vi "Read.vi"(8 "error in (no error)":errorcluster, 11 "WebSocket in":refnum<class "WebSocket.lvclass">) -> (0 "error out":errorcluster, 3 "WebSocket out":refnum<class "WebSocket.lvclass">)   [LabVIEW 2021, in "WebSocket.lvlib" / "WebSocket.lvclass"]
uses:
  WebSocket.lvclass
  C:/Program Files (x86)/National Instruments/LabVIEW 2021/vi.lib/ActorFramework/Actor/Actor.lvclass
  WebSocket.lvclass/WebSocket.ctl
  <vilib>/ActorFramework/Actor/Actor.lvclass/Actor.ctl
  <vilib>/ActorFramework/Message Enqueuer/Message Enqueuer.lvclass/Message Enqueuer.ctl
  <vilib>/ActorFramework/Message Enqueuer/Init from Existing Queue.vi
  <vilib>/ActorFramework/Message Enqueuer/Enqueue.vi
  WebSocket Messages/Read Msg/Read Msg.lvclass
  C:/Program Files (x86)/National Instruments/LabVIEW 2021/vi.lib/ActorFramework/Message/Message.lvclass
  WebSocket Messages/WaitListener Msg/WaitListener Msg.lvclass
  <vilib>/ActorFramework/Message Priority Queue/Priority Enqueue.vi
  <vilib>/ActorFramework/Message Enqueuer/Message Enqueuer.lvclass
  <vilib>/MediaMongrels Ltd/WebSockets/WebSockets/WebSocket Server/WebSocket Server.lvclass
  <vilib>/ActorFramework/Actor/Actor.lvclass
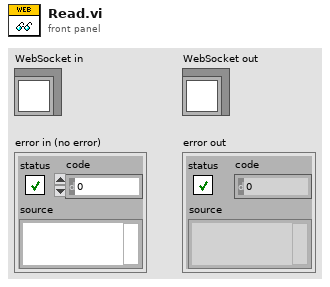
[diagram p1: front panel]
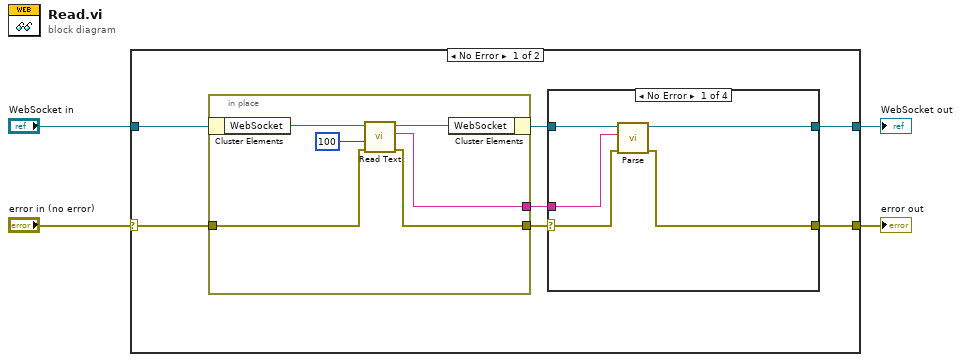
[diagram p0: block diagram]
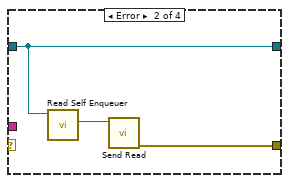
[diagram p2: hidden frame]
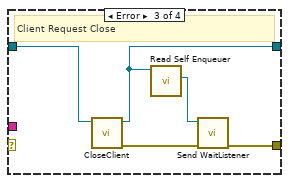
[diagram p3: hidden frame]
diagram:
  n1 = case shown="No Error" "error in (no error)" {
    selector: "error in (no error)" -> [w10 w34]
    tunnel: [w5 w34] -> w3
    tunnel: [w8 w33] -> w1
    tunnel: "WebSocket in" -> [w11 w33]
    frame No Error {
      n2 = in-place {
        in-place-border: w10 -> [w29]
        in-place-border: [w28] -> w6
        in-place-border: [w27] -> w7
        n3 = in-place-cluster #1(w11) -> ("WebSocket"=w31:refnum<class "WebSocket Server.lvclass">)
        n4 = call-dynamic "Read Text.vi"("error in (no error)"=w29, "timeout ms (5000)"=100 ("timeout ms (25000)"), "WebSocket in"=w31) -> ("error out"=w28:errorcluster, "Data"=w27:string, "WebSocket out"=w30:refnum<class "WebSocket Server.lvclass">)  [unwired: 6 in]
        n5 = in-place-cluster #1("WebSocket"=w30) -> (w9:refnum<class "WebSocket.lvclass">)
      }
      n6 = case shown="No Error" w6 {
        selector: w6 -> [w12 _ _ w25]
        tunnel: w9 -> [w16 w19 w24 w26]
        tunnel: [w15 w19 w20 w26] -> w8
        tunnel: w7 -> [w14 _ _ _]
        tunnel: [w13 w17 w21 w25] -> w5
        frame No Error {
          n7 = call "Parse.vi"("error in (no error)"=w12, "Data"=w14, "WebSocket in"=w16) -> ("error out"=w13:errorcluster, "WebSocket out"=w15:refnum<class "WebSocket.lvclass">)  [unwired: 7 in]
        }
        frame Error {
          n8 = call <vilib>:"Read Self Enqueuer.vi"("Actor"=w19) -> ("Self Enqueuer"=w18:refnum<class "Message Enqueuer.lvclass">)  [unwired: 10 in]
          n9 = call "Send Read.vi"("Message Enqueuer"=w18) -> ("error out"=w17:errorcluster)  [unwired: 9 in, 1 out]
        }
        frame Error {
          # "Client Request Close"
          n10 = call "CloseClient.vi"("WebSocket in"=w24) -> ("error out"=w22:errorcluster, "WebSocket out"=w20:refnum<class "WebSocket.lvclass">)  [unwired: 9 in]
          n11 = call <vilib>:"Read Self Enqueuer.vi"("Actor"=w20) -> ("Self Enqueuer"=w23:refnum<class "Message Enqueuer.lvclass">)  [unwired: 10 in]
          n12 = call "Send WaitListener.vi"("error in (no error)"=w22, "Message Enqueuer"=w23) -> ("error out"=w21:errorcluster)  [unwired: 8 in, 1 out]
        }
        frame Default {
        }
      }
    }
    frame Error {
    }
  }
  "error out" <- w3
  "WebSocket out" <- w1
